vi "VisualizePMU.vi"() -> ()   [LabVIEW 2017, in "Visualization.lvlib" / "VisualizePMU_class.lvclass"]
uses:
  VisualizePMU_class.lvclass
  Framework/Bus_class/Bus.lvclass
  VisializeBase_class/Typedefs/VisualizeData.ctl
  VisializeBase_class/Typedefs/clVisualizeData.ctl
  Modules/EventPlugins/EventPluginBaseClass/TypeDefs/clEvtReportArray.ctl
  Modules/EventPlugins/EventPluginBaseClass/TypeDefs/clEvtReport.ctl
  Modules/EventPlugins/EventPluginBaseClass/TypeDefs/dblEvtSignalArray.ctl
  Modules/NetworkImpairmentModule/PublicAPI/Arguments/Broadcasts/dblNetworkTime.ctl
  Modules/NetworkImpairmentModule/PublicAPI/Arguments/Broadcasts/dblPktLoss.ctl
  Modules/FlagImpairModule/PublicAPI/Arguments/Broadcasts/ui32FlagImpairmentArray.ctl
  Framework/Bus_class/Broadcast/Typedefs/clDidInit.ctl
  QMH/Typedefs/clEvtRptArray.ctl
  QMH/Typedefs/clEvtRptSignal.ctl
  QMH/Typedefs/clPmuImpairRptArray.ctl
  VisializeBase_class/Requests/clUserEventType.ctl
  <vilib>/event_ctls.llb/usereventprio.ctl
  <vilib>/Utility/miscctls.llb/LVStringsAndValuesArrayTypeDef_U8.ctl
  QMH/Typedefs/clNetImpairmentTime.ctl
  QMH/Typedefs/clNetIPktLoss.ctl
  QMH/Typedefs/clFlagImpairArray.ctl
  <vilib>/Utility/error.llb/Error Cluster From Error Code.vi
  <vilib>/ErrorRing/Error Ring.xnode
  VisializeBase_class/VisualizeBase_class.lvclass
  <userlib>/NIST/NISTErrorLib/NISTErrorLib.lvlib
  Framework/Bus_class/Bus_class.lvlib
  Modules/EventModule/EventModule.lvlib
  Modules/PmuImpairModule/PmuImpairModule.lvlib
  Modules/NetworkImpairmentModule/NetworkImpairmentModule.lvlib
  Modules/FlagImpairModule/FlagImpairModule.lvlib
  Modules/EventPlugins/EventPluginBaseClass/EventPluginBaseClass.lvclass
  VisualizeApp_class/VisualizeAppBase_class.lvclass
panel:
  in  "QueName":string="VisPmuQue"
  out "RFE Plot":cluster{dbl[], "TVE":dbl[]}[](graph)
  out "FE Plot":cluster{dbl[], "TVE":dbl[]}[](graph)
  out "PE Plot":cluster{dbl[], "TVE":dbl[]}[](graph)
  out "Mag Error":cluster{dbl[], "TVE":dbl[]}[](graph)
  out "TVE Plot":cluster{dbl[], "TVE":dbl[]}[](graph)
  in  "Bus Number":u8(ring)
  out "ErrorArray":errorcluster[](array[cluster])
  in  "btnStop":bool
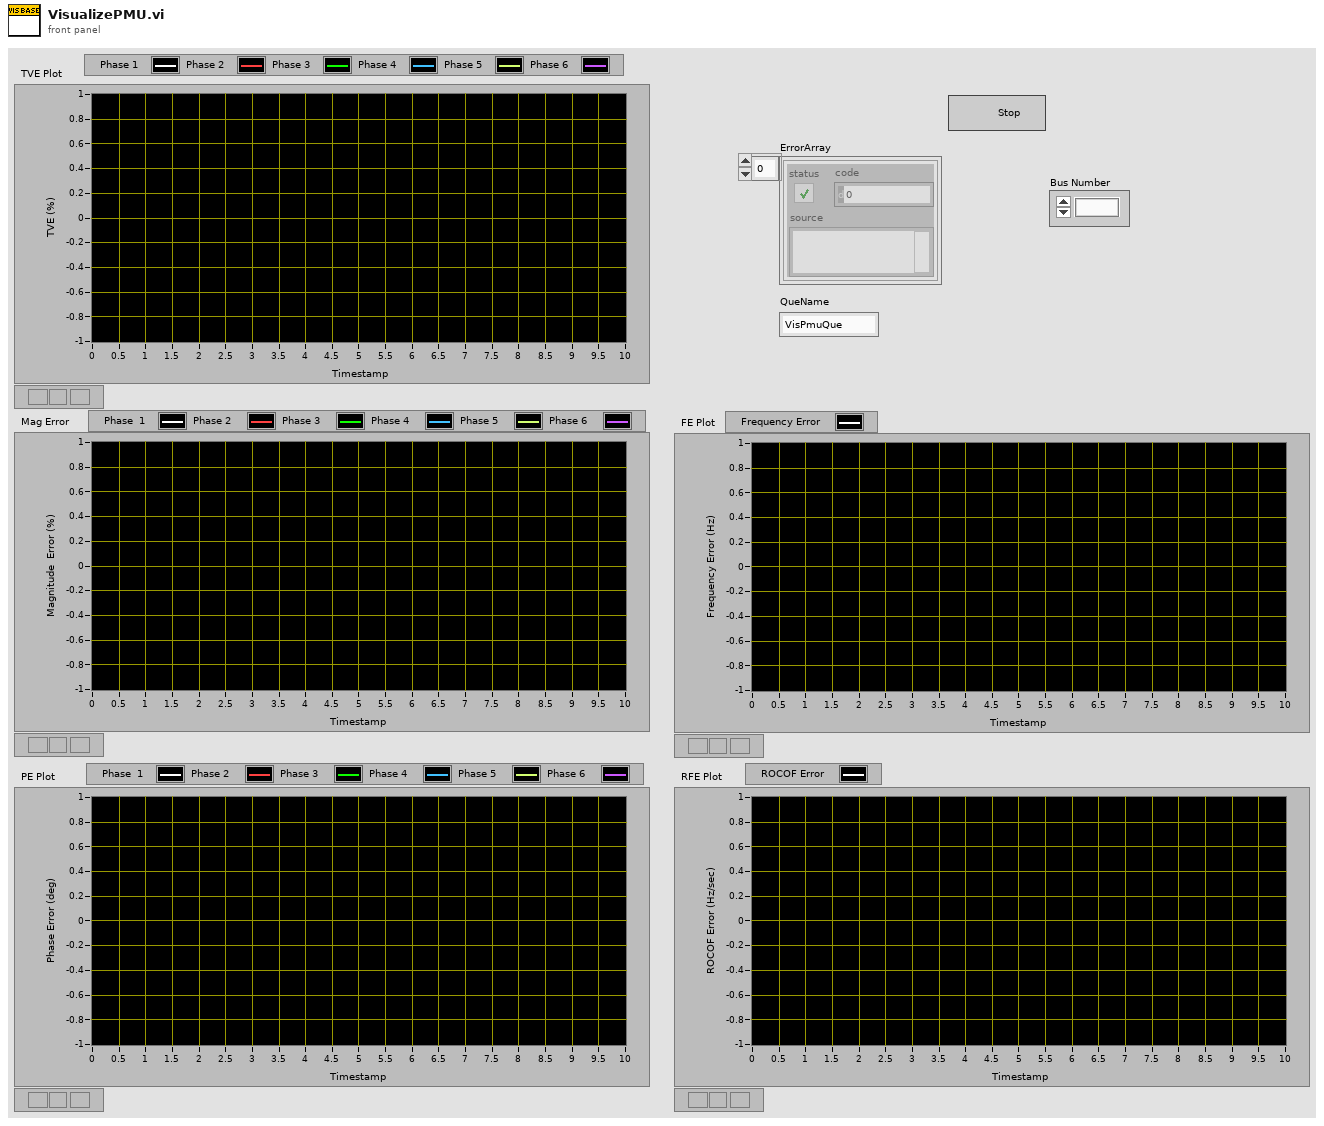
[diagram p1: front panel]
types:
  T1 = typedef "Visualization.lvlib/VisualizeBase_class.lvclass/VisualizeData.ctl" = T2[]
  T2 = typedef "Visualization.lvlib/VisualizeAppBase_class.lvclass/clVisualizeData.ctl" = cluster{"clEvtReportArray":T3, "dblEventSignalArray":T5, "clPmuImpairRptArray":T3, "dblNetworkTime":T6, "dblPktLoss":T7, "FlagImpairArray":T8, "TimeArray":dbl[]}
  T3 = typedef "EventPlugins.lvlib/EventPluginBaseClass.lvclass/clEvtReportArray.ctl" = T4[]
  T4 = typedef "EventPlugins.lvlib/EventPluginBaseClass.lvclass/clEvtReport.ctl" = cluster{"Timestamp":dbl, "Synx":cdb[], "Freq":dbl, "ROCOF":dbl, "ID":i16}
  T5 = typedef "EventPlugins.lvlib/EventPluginBaseClass.lvclass/dblEvtSignalArray.ctl" = dbl[][]
  T6 = typedef "NetworkImpairmentModule.lvlib/dblNetworkTime.ctl" = dbl[]
  T7 = typedef "NetworkImpairmentModule.lvlib/dblPktLoss.ctl" = dbl[]
  T8 = typedef "FlagImpairModule.lvlib/ui32FlagImpairmentArray.ctl" = u32[]
  T9 = typedef "Visualization.lvlib/VisualizeBase_class.lvclass/clRequestEvents.ctl" = cluster{"StopRequest":refnum<user-event>}
  T10 = typedef "Bus_class.lvlib/clBroadcastEvents.ctl" = cluster{"DidInit":refnum<user-event>, "DidStop":refnum<user-event>}
  T11 = typedef "EventModule.lvlib/clBroadcastEvents.ctl" = cluster{"DidInit":refnum<user-event>, "StatusUpdate":refnum<user-event>, "ErrorReport":refnum<user-event>, "DidStop":refnum<user-event>, "ReadEvtConfig":refnum<user-event>, "ReadTimeArray":refnum<user-event>, "ReadEvtParams":refnum<user-event>, "GetEvtReportArray":refnum<user-event>, "ReadPathToPlugin":refnum<user-event>, "GetEvtSignal":refnum<user-event>, "ReadBusNumber":refnum<user-event>}
  T12 = typedef "PmuImpairModule.lvlib/clBroadcastEvents.ctl" = cluster{"DidInit":refnum<user-event>, "StatusUpdate":refnum<user-event>, "ErrorReport":refnum<user-event>, "DidStop":refnum<user-event>, "ImpairConfig":refnum<user-event>, "ImpairParams":refnum<user-event>, "ImpairReports":refnum<user-event>, "PathToPlugin":refnum<user-event>, "BusNumber":refnum<user-event>}
  T13 = typedef "NetworkImpairmentModule.lvlib/clBroadcastEvents.ctl" = cluster{"DidInit":refnum<user-event>, "StatusUpdate":refnum<user-event>, "ErrorReport":refnum<user-event>, "DidStop":refnum<user-event>, "ReadNetImpParams":refnum<user-event>, "ReadLossThreshold":refnum<user-event>, "GetNetworkTime":refnum<user-event>, "GetPktLoss":refnum<user-event>, "ReadPathToPlugin":refnum<user-event>}
  T14 = typedef "FlagImpairModule.lvlib/clBroadcastEvents.ctl" = cluster{"DidInit":refnum<user-event>, "StatusUpdate":refnum<user-event>, "ErrorReport":refnum<user-event>, "DidStop":refnum<user-event>, "ReadFlagImpairConfig":refnum<user-event>, "ReadPluginINIFilePath":refnum<user-event>, "ReadFlagImpairParams":refnum<user-event>, "ReadTimeArray":refnum<user-event>, "GetFlagImpairment":refnum<user-event>}
  T15 = cluster{"BusNumberRef":refnum<vi>, "TVE Plot":refnum<vi>, "Mag Error":refnum<vi>, "PE Plot":refnum<vi>, "FE Plot":refnum<vi>, "RFE Plot":refnum<vi>}
  T16 = typedef "LVStringsAndValuesArrayTypeDef_U8.ctl" = cluster{"String":string, "Value":u8}[]
  T17 = typedef "Visualization.lvlib/VisualizeBase_class.lvclass/clEvtRptArray.ctl" = cluster{"BusIndex":i32, "clImpairReportArray":T3}
  T18 = typedef "Visualization.lvlib/VisualizeBase_class.lvclass/clPmuImpairRptArray.ctl" = cluster{"BusIndex":i32, "clImpairReportArray":T3}
  T19 = typedef "Visualization.lvlib/VisualizeBase_class.lvclass/clNetImpairmentTime.ctl" = cluster{"BusIndex":i32, "clNetImpairTimeArray":T6}
  T20 = typedef "Visualization.lvlib/VisualizeBase_class.lvclass/clNetIPktLoss.ctl" = cluster{"BusIndex":i32, "clNetPktLoss":T7}
  T21 = typedef "Visualization.lvlib/VisualizeBase_class.lvclass/clFlagImpairArray.ctl" = cluster{"BusIndex":i32, "FlagImpairArray":T8}
  T22 = typedef "Visualization.lvlib/VisualizeBase_class.lvclass/clEvtRptSignal.ctl" = cluster{"BusIndex":i32, "dblEventSignalArray":T5}
  T23 = typedef "Visualization.lvlib/VisualizeBase_class.lvclass/clUserEventType.ctl" = cluster{"BusIndex":i8, "Data":variant}
  T24 = typedef "usereventprio.ctl" = enum32{"high priority", "normal priority"}
  T25 = typedef "Bus_class.lvlib/clDidInit.ctl" = cluster{"Bus":refnum<vi>, "Init?":bool}
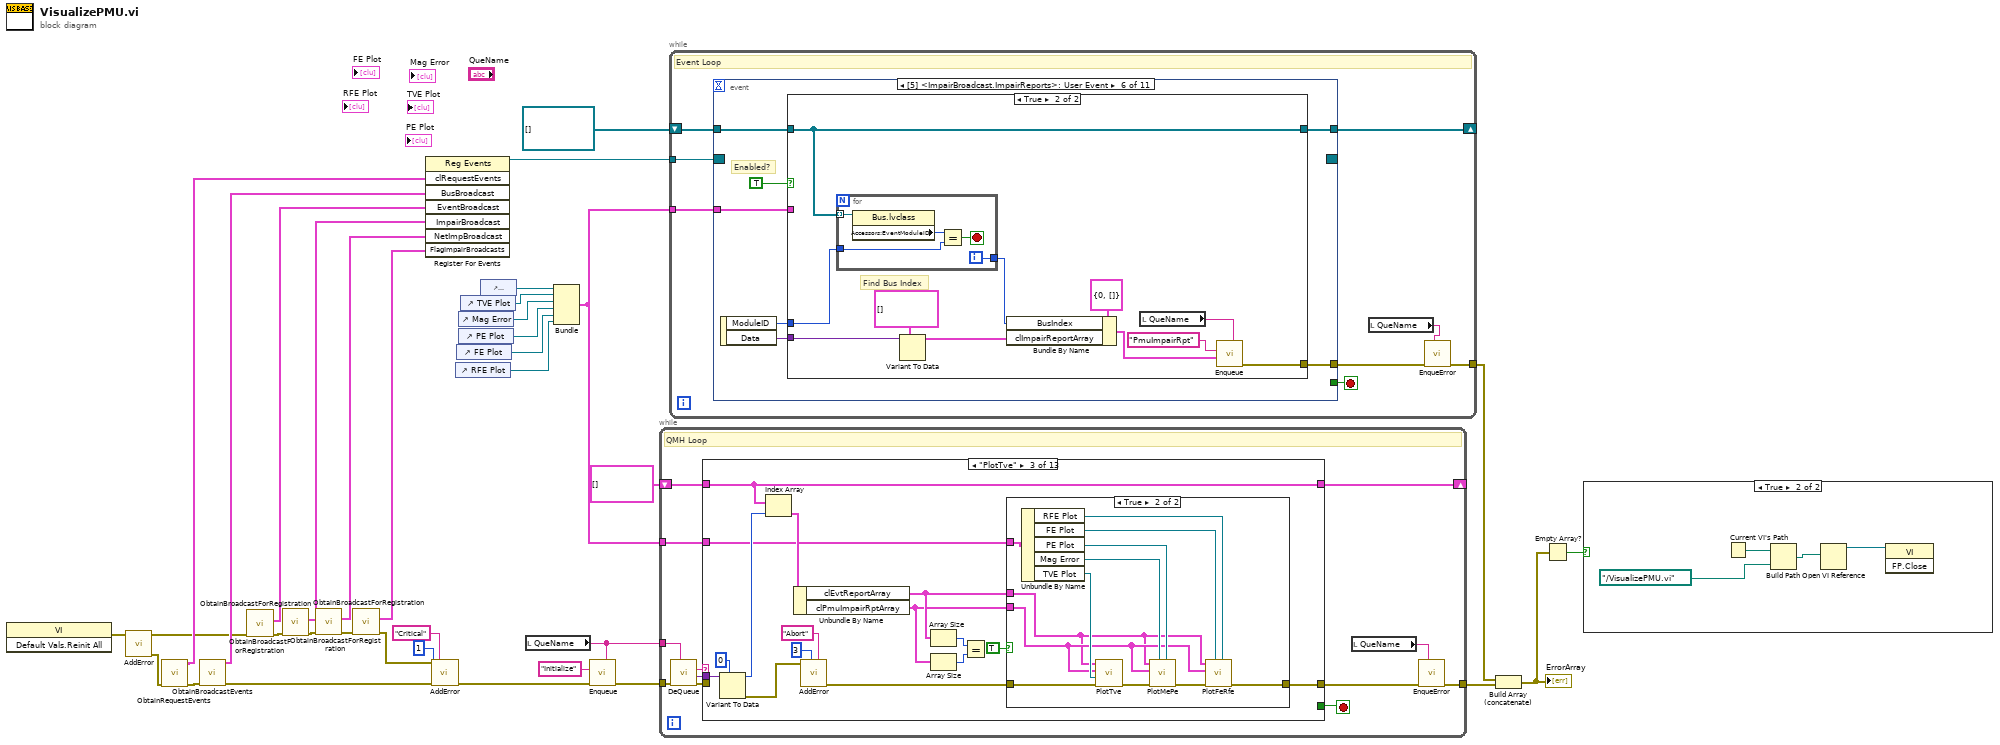
[diagram p0: block diagram]
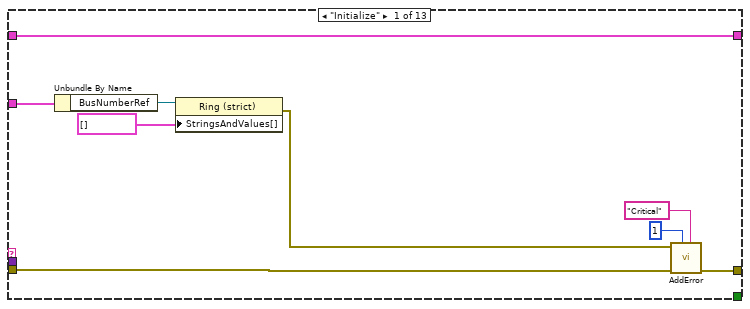
[diagram p3: hidden frame]
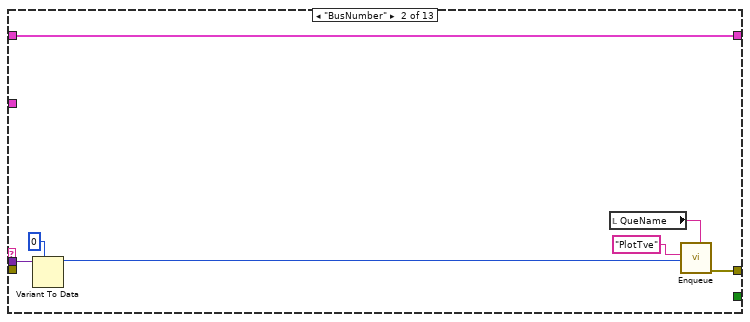
[diagram p4: hidden frame]
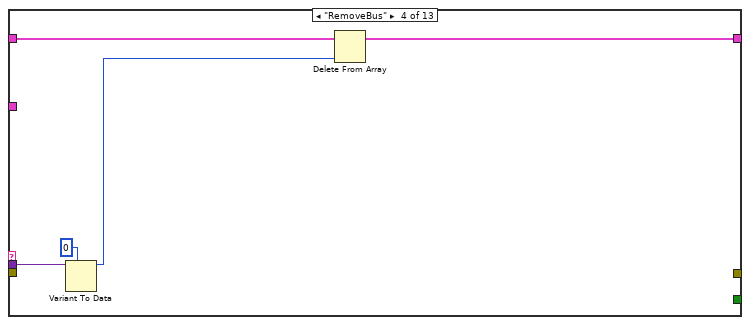
[diagram p6: hidden frame]
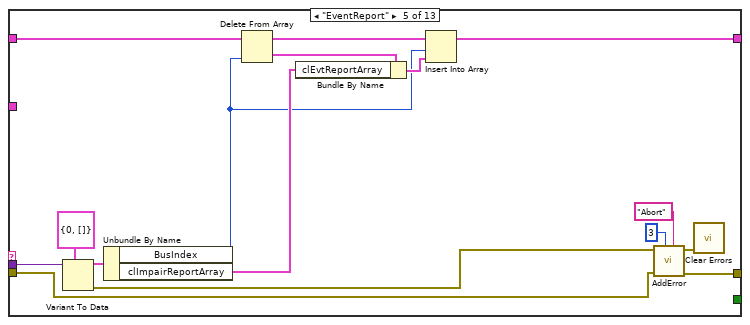
[diagram p7: hidden frame]
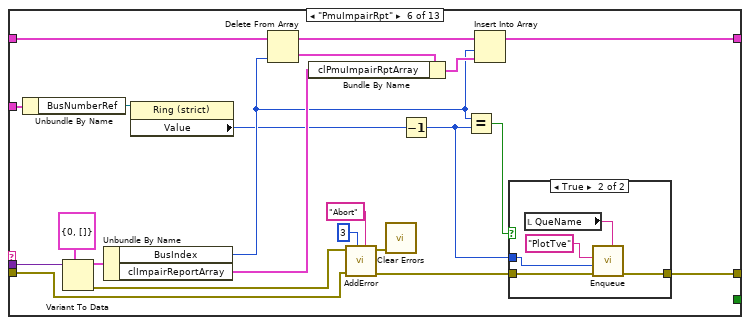
[diagram p8: hidden frame]
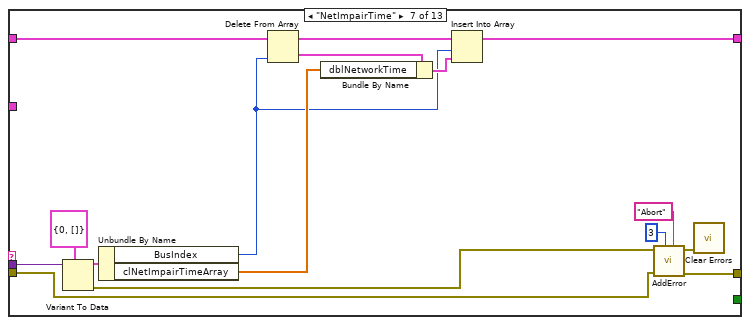
[diagram p10: hidden frame]
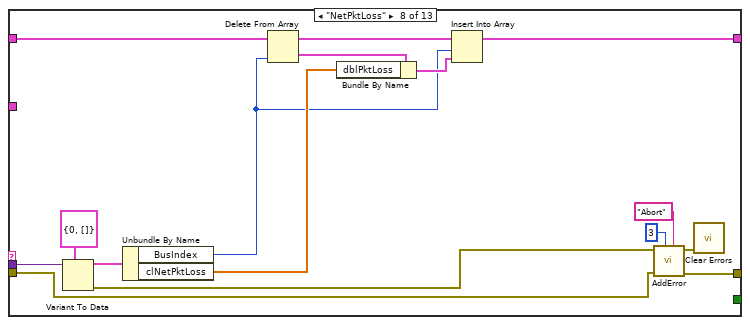
[diagram p11: hidden frame]
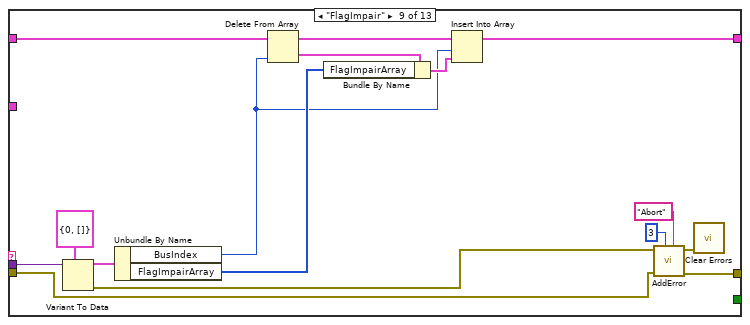
[diagram p12: hidden frame]
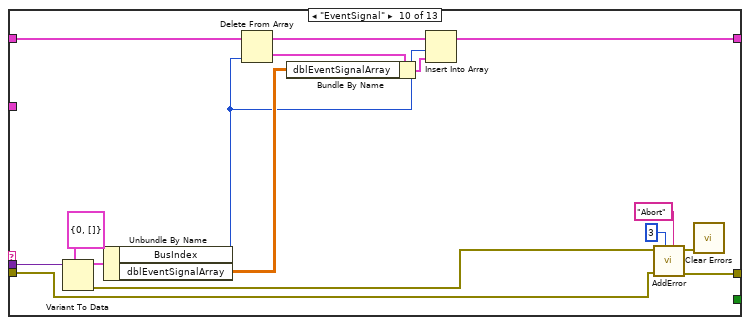
[diagram p13: hidden frame]
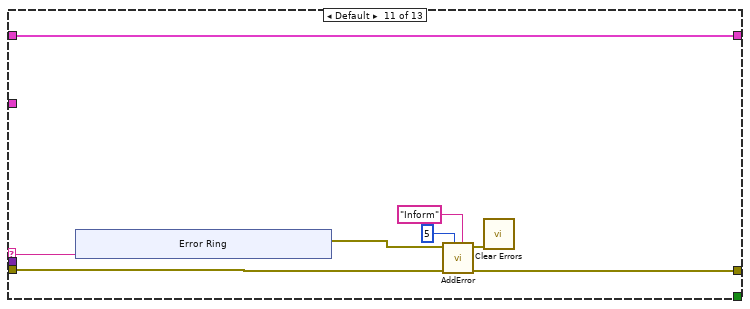
[diagram p14: hidden frame]
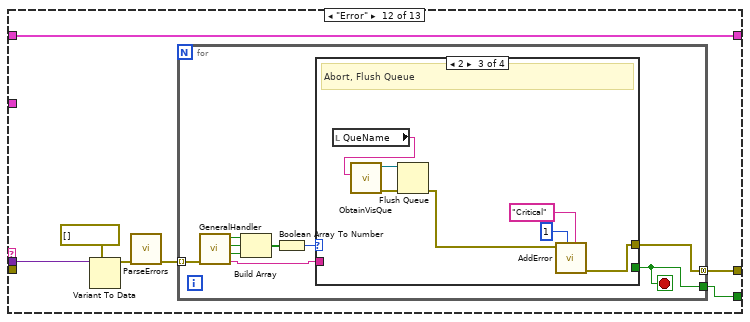
[diagram p15: hidden frame]
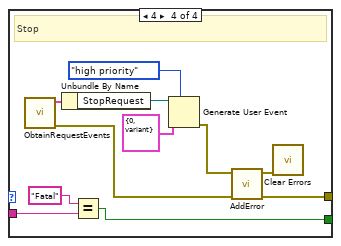
[diagram p18: hidden frame]
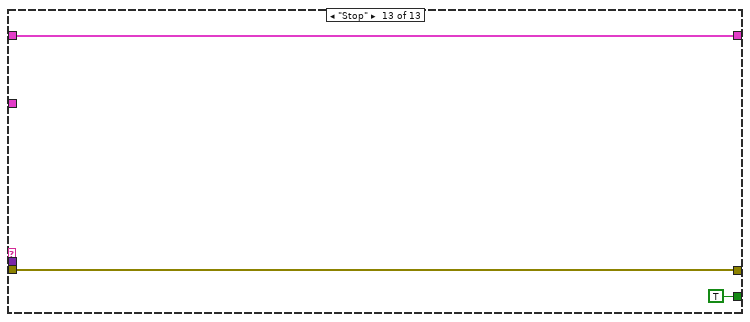
[diagram p19: hidden frame]
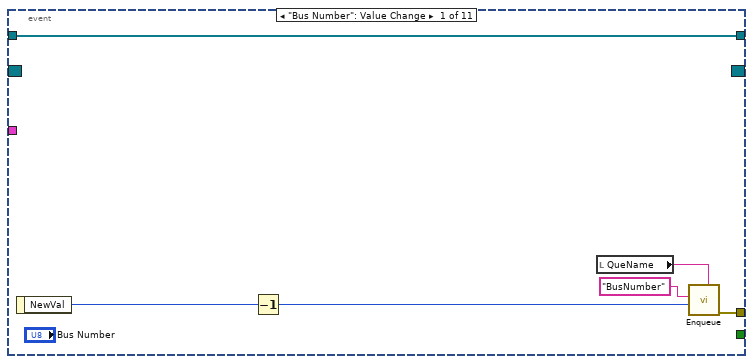
[diagram p20: hidden frame]
diagram:
  n1 = invoke class="VI" method="Default Vals.Reinit All"() -> (error out=w25:errorcluster)  [unwired: 3 in, 2 out]
  n2 = call <userlib>:"AddError.vi"("error in (no error)"=w25) -> ("ErrorArray"=w24:errorcluster[], "error out"=w16:errorcluster)  [unwired: 9 in]
  n3 = call "ObtainRequestEvents.vi"("Error"=w24) -> ("Error"=w29:errorcluster[], "clRequestEvents"=w33:T9)  [unwired: 9 in]
  n4 = call "ObtainBroadcastEvents.vi"("ErrorArray"=w29) -> ("ErrorArray"=w15:errorcluster[], "BusBroadcast"=w28:T10)  [unwired: 9 in]
  n5 = call "ObtainBroadcastForRegistration.vi"("error in (no error)"=w16) -> ("error out"=w19:errorcluster, "EventBroadcast"=w23:T11)  [unwired: 9 in]
  n6 = call "ObtainBroadcastForRegistration.vi"("error in (no error)"=w19) -> ("error out"=w18:errorcluster, "ImpairBroadcast"=w22:T12)  [unwired: 9 in]
  n7 = call "ObtainBroadcastForRegistration.vi"("error in (no error)"=w18) -> ("error out"=w17:errorcluster, "NetImpBroadcast"=w21:T13)  [unwired: 9 in]
  n8 = call "ObtainBroadcastForRegistration.vi"("error in (no error)"=w17) -> ("error out"=w14:errorcluster, "FlagImpairBroadcasts"=w20:T14)  [unwired: 9 in]
  n9 = register-events(w33, w28, w23, w22, w21, w20) -> (reference out=w32:refnum<event-registration>)  [unwired: 2 in, 1 out]
  n10 = call <userlib>:"AddError.vi"("Severity"="Critical" ("String"), "Priority"=u8 1, "ErrorArray"=w15, "error in (no error)"=w14) -> ("ErrorArray"=w11:errorcluster[])  [unwired: 6 in, 1 out]
  n11 = control-ref of="RFE Plot"() -> (w4:refnum<vi>)
  n12 = control-ref of="FE Plot"() -> (w5:refnum<vi>)
  n13 = control-ref of="PE Plot"() -> (w6:refnum<vi>)
  n14 = control-ref of="Mag Error"() -> (w7:refnum<vi>)
  n15 = control-ref of="TVE Plot"() -> (w8:refnum<vi>)
  n16 = control-ref of="BusNumberRef"() -> (w27:refnum<vi>)
  n17 = local read "QueName"() -> (w3:string)
  n18 = Bundle("BusNumberRef"=w27, "TVE Plot"=w8, "Mag Error"=w7, "PE Plot"=w6, "FE Plot"=w5, "RFE Plot"=w4) -> (w9:T15)  [unwired: 1 in]
  n19 = call "Enqueue.vi"("QueName"=w3, "Error"=w11, "Message"="Initialize") -> ("Error"=w34:errorcluster[])  [unwired: 8 in]
  n20 = while {
    tunnel: w34 -> [w47]
    tunnel: [w41] -> w31
    tunnel: w9 -> [w40]
    shift-right: [w38] -> _
    shift-left: T1 [] ("VisualizeData") -> [w39]
    tunnel: w3 -> [w36]
    stop <- w42 stop-if-true
    # "QMH Loop"
    n21 = call "DeQueue.vi"("QueName"=w36, "Error"=w47) -> ("Error"=w44:errorcluster[], "Data"=w45:variant, "Message"=w46:string)  [unwired: 7 in]
    n22 = case shown="\"PlotTve\"" w46 {
      selector: w46 -> [_ _ _ _ _ _ _ _ _ _ w212 _ _]
      tunnel: w45 -> [_ w61 w79 w96 w112 w134 w156 w172 w188 w204 _ w226 _]
      tunnel: w44 -> [w53 _ _ _ w97 w121 w141 w157 w173 w189 w210 _ w255]
      tunnel: [w52 w63 w69 _ w102 w119 w146 w162 w178 w194 w209 w222 w255] -> w43
      tunnel: [_ _ _ _ _ _ _ _ _ _ _ w221 TRUE] -> w42
      tunnel: w40 -> [w56 _ w72 _ _ w118 _ _ _ _ _ _ _]
      tunnel: w39 -> [w48 w58 w77 w94 w108 w130 w152 w168 w184 w200 w205 w220 w254]
      tunnel: [w48 w58 w77 w93 w109 w131 w153 w169 w185 w201 w205 w220 w254] -> w38
      frame "Initialize" {
        n23 = Unbundle By Name(w56) -> ("BusNumberRef"=w55:refnum<vi>)
        n24 = property class="Ring (strict)"(reference=w55, "StringsAndValues[]"=T16 [] ("Strings And Values []")) -> (error out=w51:errorcluster)  [unwired: 1 in, 1 out]
        n25 = call <userlib>:"AddError.vi"("Severity"="Critical" ("String"), "Priority"=u8 1, "ErrorArray"=w53, "error in (no error)"=w51) -> ("ErrorArray"=w52:errorcluster[])  [unwired: 6 in, 1 out]
      }
      frame "BusNumber" {
        n26 = Variant To Data(type=u8 0 ("NewVal"), Variant=w61) -> (data=w60:u8)  [unwired: 1 in, 1 out]
        n27 = local read "QueName"() -> (w57:string)
        n28 = call "Enqueue.vi"("QueName"=w57, "Data"=w60, "Message"="PlotTve") -> ("Error"=w63:errorcluster[])  [unwired: 8 in]
      }
      frame "PlotTve" {
        n29 = Variant To Data(type=u8 0 ("NewVal"), Variant=w79) -> (data=w76:u8, error out=w68:errorcluster)  [unwired: 1 in]
        n30 = Index Array(array=w77, index=w76) -> (element=w75:T2)
        n31 = Unbundle By Name(w75) -> ("clEvtReportArray"=w71:T3, "clPmuImpairRptArray"=w70:T3)
        n32 = call <userlib>:"AddError.vi"("Severity"="Abort" ("String"), "Priority"=u8 3, "error in (no error)"=w68) -> ("ErrorArray"=w67:errorcluster[])  [unwired: 7 in, 1 out]
        n33 = Array Size(array=w71) -> (size(s)=w73:i32)
        n34 = Array Size(array=w70) -> (size(s)=w74:i32)
        n35 = Equal?(x=w73, y=w74) -> ()  [unwired: 1 out]
        n36 = case shown="True" TRUE {
          tunnel: w72 -> [_ w91]
          tunnel: w71 -> [_ w82]
          tunnel: w70 -> [_ w83]
          tunnel: [_ w84] -> w69
          tunnel: w67 -> [_ w89]
          frame False {
          }
          frame True {
            n37 = Unbundle By Name(w91) -> ("RFE Plot"=w80:refnum<vi>, "FE Plot"=w81:refnum<vi>, "PE Plot"=w86:refnum<vi>, "Mag Error"=w87:refnum<vi>, "TVE Plot"=w90:refnum<vi>)
            n38 = call "PlotTve.vi"("ErrorArray"=w89, "TvePlotRef"=w90, "clPMUImpairRptArray"=w83, "clEvtReportArray"=w82) -> ("ErrorArray"=w88:errorcluster[])  [unwired: 7 in]
            n39 = call "PlotMePe.vi"("PePlotRef"=w86, "MePlotRef"=w87, "ErrorArray"=w88, "clPmuRptArray"=w83, "clEvtReportArray"=w82) -> ("ErrorArray"=w85:errorcluster[])  [unwired: 6 in]
            n40 = call "PlotFeRfe.vi"("REPlotRef"=w80, "FEPlotRef"=w81, "ErrorArray"=w85, "clPmuImpairRptArray"=w83, "clEvtReportArray"=w82) -> ("ErrorArray"=w84:errorcluster[])  [unwired: 6 in]
          }
        }
      }
      frame "RemoveBus" {
        n41 = Variant To Data(type=0, Variant=w96) -> (data=w92:i32)  [unwired: 1 in, 1 out]
        n42 = Delete From Array(array=w94, index=w92) -> (array with subset deleted=w93:T1)  [unwired: 1 in, 1 out]
      }
      frame "EventReport" {
        n43 = Variant To Data(type=T17 {"BusIndex"=0, "clImpairReportArray"=[]} ("clEvtReportArray"), Variant=w112) -> (data=w110:T17, error out=w101:errorcluster)  [unwired: 1 in]
        n44 = Unbundle By Name(w110) -> ("BusIndex"=w103:i32, "clImpairReportArray"=w105:T3)
        n45 = Delete From Array(array=w108, index=w103) -> (deleted portion=w106:T2, array with subset deleted=w107:T1)  [unwired: 1 in]
        n46 = Bundle By Name(cluster=w106, "clEvtReportArray"=w105) -> (w104:T2)
        n47 = Insert Into Array(array=w107, index=w103, new element=w104) -> (w109:T1)
        n48 = call <userlib>:"AddError.vi"("Severity"="Abort" ("String"), "Priority"=u8 3, "ErrorArray"=w97, "error in (no error)"=w101) -> ("ErrorArray"=w102:errorcluster[], "error out"=w100:errorcluster)  [unwired: 6 in]
        n49 = call <vilib>:"Clear Errors.vi"("error in (no error)"=w100) -> ()  [unwired: 5 in, 2 out]
      }
      frame "PmuImpairRpt" {
        n50 = Unbundle By Name(w118) -> ("BusNumberRef"=w117:refnum<vi>)
        n51 = Variant To Data(type=T18 {"BusIndex"=0, "clImpairReportArray"=[]} ("clImpairReportArray"), Variant=w134) -> (data=w132:T18, error out=w125:errorcluster)  [unwired: 1 in]
        n52 = Unbundle By Name(w132) -> ("BusIndex"=w116:i32, "clImpairReportArray"=w127:T3)
        n53 = property class="Ring (strict)"(reference=w117) -> ("Value"=w114:u8)  [unwired: 1 in, 2 out]
        n54 = Delete From Array(array=w130, index=w116) -> (deleted portion=w128:T2, array with subset deleted=w129:T1)  [unwired: 1 in]
        n55 = Bundle By Name(cluster=w128, "clPmuImpairRptArray"=w127) -> (w126:T2)
        n56 = call <userlib>:"AddError.vi"("Severity"="Abort" ("String"), "Priority"=u8 3, "ErrorArray"=w121, "error in (no error)"=w125) -> ("ErrorArray"=w120:errorcluster[], "error out"=w124:errorcluster)  [unwired: 6 in]
        n57 = call <vilib>:"Clear Errors.vi"("error in (no error)"=w124) -> ()  [unwired: 5 in, 2 out]
        n58 = Decrement(x=w114) -> (x-1=w113:u8)
        n59 = Equal?(x=w116, y=w113) -> (x = y?=w115:bool)
        n60 = Insert Into Array(array=w129, index=w116, new element=w126) -> (w131:T1)
        n61 = case shown="True" w115 {
          tunnel: w120 -> [w135 w140]
          tunnel: [w135 w139] -> w119
          tunnel: w113 -> [_ w137]
          frame False {
          }
          frame True {
            n62 = local read "QueName"() -> (w136:string)
            n63 = call "Enqueue.vi"("QueName"=w136, "Error"=w140, "Data"=w137, "Message"="PlotTve") -> ("Error"=w139:errorcluster[])  [unwired: 7 in]
          }
        }
      }
      frame "NetImpairTime" {
        n64 = Variant To Data(type=T19 {"BusIndex"=0, "clNetImpairTimeArray"=[]} ("clImpairReportArray"), Variant=w156) -> (data=w154:T19, error out=w145:errorcluster)  [unwired: 1 in]
        n65 = Unbundle By Name(w154) -> ("BusIndex"=w147:i32, "clNetImpairTimeArray"=w149:T6)
        n66 = Delete From Array(array=w152, index=w147) -> (deleted portion=w150:T2, array with subset deleted=w151:T1)  [unwired: 1 in]
        n67 = Bundle By Name(cluster=w150, "dblNetworkTime"=w149) -> (w148:T2)
        n68 = Insert Into Array(array=w151, index=w147, new element=w148) -> (w153:T1)
        n69 = call <userlib>:"AddError.vi"("Severity"="Abort" ("String"), "Priority"=u8 3, "ErrorArray"=w141, "error in (no error)"=w145) -> ("ErrorArray"=w146:errorcluster[], "error out"=w144:errorcluster)  [unwired: 6 in]
        n70 = call <vilib>:"Clear Errors.vi"("error in (no error)"=w144) -> ()  [unwired: 5 in, 2 out]
      }
      frame "NetPktLoss" {
        n71 = Variant To Data(type=T20 {"BusIndex"=0, "clNetPktLoss"=[]} ("clNetPktLoss"), Variant=w172) -> (data=w170:T20, error out=w161:errorcluster)  [unwired: 1 in]
        n72 = Unbundle By Name(w170) -> ("BusIndex"=w163:i32, "clNetPktLoss"=w165:T7)
        n73 = Delete From Array(array=w168, index=w163) -> (deleted portion=w166:T2, array with subset deleted=w167:T1)  [unwired: 1 in]
        n74 = Bundle By Name(cluster=w166, "dblPktLoss"=w165) -> (w164:T2)
        n75 = Insert Into Array(array=w167, index=w163, new element=w164) -> (w169:T1)
        n76 = call <userlib>:"AddError.vi"("Severity"="Abort" ("String"), "Priority"=u8 3, "ErrorArray"=w157, "error in (no error)"=w161) -> ("ErrorArray"=w162:errorcluster[], "error out"=w160:errorcluster)  [unwired: 6 in]
        n77 = call <vilib>:"Clear Errors.vi"("error in (no error)"=w160) -> ()  [unwired: 5 in, 2 out]
      }
      frame "FlagImpair" {
        n78 = Variant To Data(type=T21 {"BusIndex"=0, "FlagImpairArray"=[]} ("clFlagImpairArray"), Variant=w188) -> (data=w186:T21, error out=w177:errorcluster)  [unwired: 1 in]
        n79 = Unbundle By Name(w186) -> ("BusIndex"=w179:i32, "FlagImpairArray"=w181:T8)
        n80 = Delete From Array(array=w184, index=w179) -> (deleted portion=w182:T2, array with subset deleted=w183:T1)  [unwired: 1 in]
        n81 = Bundle By Name(cluster=w182, "FlagImpairArray"=w181) -> (w180:T2)
        n82 = Insert Into Array(array=w183, index=w179, new element=w180) -> (w185:T1)
        n83 = call <userlib>:"AddError.vi"("Severity"="Abort" ("String"), "Priority"=u8 3, "ErrorArray"=w173, "error in (no error)"=w177) -> ("ErrorArray"=w178:errorcluster[], "error out"=w176:errorcluster)  [unwired: 6 in]
        n84 = call <vilib>:"Clear Errors.vi"("error in (no error)"=w176) -> ()  [unwired: 5 in, 2 out]
      }
      frame "EventSignal" {
        n85 = Variant To Data(type=T22 {"BusIndex"=0, "dblEventSignalArray"=[]} ("clEvtReportArray"), Variant=w204) -> (data=w202:T22, error out=w193:errorcluster)  [unwired: 1 in]
        n86 = Unbundle By Name(w202) -> ("BusIndex"=w195:i32, "dblEventSignalArray"=w197:T5)
        n87 = Delete From Array(array=w200, index=w195) -> (deleted portion=w198:T2, array with subset deleted=w199:T1)  [unwired: 1 in]
        n88 = Bundle By Name(cluster=w198, "dblEventSignalArray"=w197) -> (w196:T2)
        n89 = Insert Into Array(array=w199, index=w195, new element=w196) -> (w201:T1)
        n90 = call <userlib>:"AddError.vi"("Severity"="Abort" ("String"), "Priority"=u8 3, "ErrorArray"=w189, "error in (no error)"=w193) -> ("ErrorArray"=w194:errorcluster[], "error out"=w192:errorcluster)  [unwired: 6 in]
        n91 = call <vilib>:"Clear Errors.vi"("error in (no error)"=w192) -> ()  [unwired: 5 in, 2 out]
      }
      frame Default {
        n92 = xnode "Error Ring"("parameter 0"=w212) -> ("error out"=w211:errorcluster)
        n93 = call <userlib>:"AddError.vi"("Severity"="Inform" ("String"), "Priority"=u8 5, "ErrorArray"=w210, "error in (no error)"=w211) -> ("ErrorArray"=w209:errorcluster[], "error out"=w208:errorcluster)  [unwired: 6 in]
        n94 = call <vilib>:"Clear Errors.vi"("error in (no error)"=w208) -> ()  [unwired: 5 in, 2 out]
      }
      frame "Error" {
        n95 = Variant To Data(type=errorcluster[] [], Variant=w226) -> (data=w224:errorcluster[])  [unwired: 1 in, 1 out]
        n96 = call <userlib>:"ParseErrors.vi"("ErrorArray"=w224) -> ("ErrorArray"=w223:errorcluster[])  [unwired: 8 in, 2 out]
        n97 = for {
          tunnel: w223 -> [w235] mode=indexing
          tunnel: [w229] -> w222 mode=concatenating
          tunnel: [w227] -> w221
          stop <- w227 stop-if-true
          n98 = call <userlib>:"GeneralHandler.vi"("error in (no error)"=w235) -> ("Severity"=w228:string, "Stop"=w232:bool, "Abort"=w233:bool, "Continue"=w234:bool)  [unwired: 7 in]
          n99 = Build Array(w234, w233, w232) -> (w231:bool[])
          n100 = Boolean Array To Number(Boolean array=w231) -> (number=w230:u32)
          n101 = case shown="2" w230 {
            tunnel: [_ _ w240 w251] -> w229
            tunnel: w228 -> [_ _ _ w245]
            tunnel: [_ _ _ w243] -> w227
            frame 0, Default {
              # "No Dialog"
            }
            frame 1 {
              # "Continue"
            }
            frame 2 {
              # "Abort, Flush Queue"
              n102 = local read "QueName"() -> (w236:string)
              n103 = call "ObtainVisQue.vi"("QueName"=w236) -> ("error out"=w242:errorcluster, "queue out"=w241:refnum<queue>)  [unwired: 9 in]
              n104 = Flush Queue(queue=w241, error in (no error)=w242) -> (error out=w239:errorcluster)  [unwired: 2 out]
              n105 = call <userlib>:"AddError.vi"("Severity"="Critical" ("String"), "Priority"=u8 1, "error in (no error)"=w239) -> ("ErrorArray"=w240:errorcluster[])  [unwired: 7 in, 1 out]
            }
            frame 4 {
              # "Stop"
              n106 = call "ObtainRequestEvents.vi"() -> ("Error"=w249:errorcluster[], "clRequestEvents"=w253:T9)  [unwired: 10 in]
              n107 = Unbundle By Name(w253) -> ("StopRequest"=w252:refnum<user-event>)
              n108 = Equal?(x="Fatal", y=w245) -> (x = y?=w243:bool)
              n109 = Generate User Event(priority (normal)=usereventprio."high priority", user event=w252, event data cluster=T23 {"BusIndex"=0, "Data"=variant} ("event data")) -> (error out=w250:errorcluster)  [unwired: 1 in, 1 out]
              n110 = call <userlib>:"AddError.vi"("ErrorArray"=w249, "error in (no error)"=w250) -> ("ErrorArray"=w251:errorcluster[], "error out"=w246:errorcluster)  [unwired: 8 in]
              n111 = call <vilib>:"Clear Errors.vi"("error in (no error)"=w246) -> ()  [unwired: 5 in, 2 out]
            }
          }
        }
      }
      frame "Stop" {
      }
    }
    n112 = local read "QueName"() -> (w37:string)
    n113 = call "EnqueError.vi"("QueName"=w37, "Error"=w43) -> ("Error"=w41:errorcluster[])  [unwired: 9 in]
  }
  n114 = while {
    tunnel: w32 -> [w264]
    tunnel: [w261] -> w30
    tunnel: w9 -> [w260]
    shift-right: [w258] -> _
    shift-left: refnum<class "Bus.lvclass">[] [] -> [w259]
    stop <- w263 stop-if-true
    # "Event Loop"
    n115 = event shown="[5] <ImpairBroadcast.ImpairReports>: User Event" {
      selector: w264 -> [_ _ _ _ _ _ _ _ _ _ _]
      dyn-events: [_ w271 _ _ _ _ _ _ _ _ _] -> _
      timeout: _ -> [_ _ _ _ _ _ _ _ _ _ _]
      tunnel: [_ _ _ _ _ _ _ _ _ TRUE _] -> w263
      tunnel: [w270 w272 w300 w307 w330 w354 w377 w400 w423 w448 w456] -> w262
      tunnel: w260 -> [_ w292 w304 _ _ w351 _ _ _ _ _]
      tunnel: w259 -> [w267 w291 w303 w310 w333 w357 w380 w403 w426 w445 w450]
      tunnel: [w267 w288 w302 w305 w328 w352 w375 w398 w421 w445 w450] -> w258
      event "Bus Number": Value Change {
        n116 = event-data() -> ("NewVal"=w269:u8)  [unwired: 1 in]
        n117 = Decrement(x=w269) -> (x-1=w265:u8)
        n118 = local read "QueName"() -> (w266:string)
        n119 = call "Enqueue.vi"("QueName"=w266, "Data"=w265, "Message"="BusNumber") -> ("Error"=w270:errorcluster[])  [unwired: 8 in]
      }
      event User Event {
        n120 = event-data() -> ("Data"=w295:variant)  [unwired: 1 in]
        n121 = Unbundle By Name(w292) -> ("BusNumberRef"=w290:refnum<vi>)
        n122 = Variant To Data(type=T25 {"Bus"=refnum, "Init?"=FALSE} ("clBusDidInit"), Variant=w295) -> (data=w293:T25)  [unwired: 1 in, 1 out]
        n123 = Unbundle By Name(w293) -> ("Bus"=w289:refnum<vi>)
        n124 = call "ObtainRequestEvents.vi"() -> ("Error"=w284:errorcluster[], "clRequestEvents"=w286:T9)  [unwired: 10 in]
        n125 = call "AddBus.vi"("BusRef"=w289, "BusNumberRef"=w290, "BusArray"=w291) -> ("BusArray"=w288:refnum<class "Bus.lvclass">[])  [unwired: 8 in]
        n126 = call "ObtainBroadcastEvents.vi"("ErrorArray"=w284) -> ("ErrorArray"=w285:errorcluster[], "BusBroadcast"=w287:T10)  [unwired: 9 in]
        n127 = call "ObtainBroadcastForRegistration.vi"() -> ("error out"=w273:errorcluster, "EventBroadcast"=w280:T11)  [unwired: 10 in]
        n128 = call "ObtainBroadcastForRegistration.vi"("error in (no error)"=w273) -> ("error out"=w274:errorcluster, "ImpairBroadcast"=w281:T12)  [unwired: 9 in]
        n129 = call "ObtainBroadcastForRegistration.vi"("error in (no error)"=w274) -> ("error out"=w275:errorcluster, "NetImpBroadcast"=w282:T13)  [unwired: 9 in]
        n130 = call "ObtainBroadcastForRegistration.vi"("error in (no error)"=w275) -> ("error out"=w279:errorcluster, "FlagImpairBroadcasts"=w283:T14)  [unwired: 9 in]
        n131 = register-events(w286, w287, w280, w281, w282, w283) -> (reference out=w271:refnum<event-registration>)  [unwired: 2 in, 1 out]
        n132 = call <userlib>:"AddError.vi"("Severity"="Critical" ("String"), "Priority"=u8 1, "ErrorArray"=w285, "error in (no error)"=w279) -> ("ErrorArray"=w272:errorcluster[], "error out"=w278:errorcluster)  [unwired: 6 in]
        n133 = call <vilib>:"Clear Errors.vi"("error in (no error)"=w278) -> ()  [unwired: 5 in, 2 out]
      }
      event User Event {
        n134 = event-data() -> ("BusNumber"=w297:i8)  [unwired: 1 in]
        n135 = Unbundle By Name(w304) -> ("BusNumberRef"=w301:refnum<vi>)
        n136 = call "RemoveBus.vi"("BusArray"=w303, "BusNumberRef"=w301, "BusNumber"=w297) -> ("BusArray"=w302:refnum<class "Bus.lvclass">[], "BusIndex"=w299:i32)  [unwired: 6 in]
        n137 = local read "QueName"() -> (w296:string)
        n138 = call "Enqueue.vi"("QueName"=w296, "Data"=w299, "Message"="RemoveBus") -> ("Error"=w300:errorcluster[])  [unwired: 8 in]
      }
      event User Event {
        # "Enabled?"
        n139 = event-data() -> ("ModuleID"=w309:i32, "Data"=w308:variant)  [unwired: 1 in]
        n140 = case shown="True" TRUE {
          tunnel: w310 -> [w311 w313]
          tunnel: w309 -> [_ w322]
          tunnel: w308 -> [_ w320]
          tunnel: [_ w317] -> w307
          tunnel: [w311 w313] -> w305
          frame False {
          }
          frame True {
            # "Find Bus Index"
            n141 = for {
              tunnel: w313 -> [w327] mode=indexing
              tunnel: w322 -> [w325]
              tunnel: [w323] -> w321
              i -> [w323]
              stop <- w324 stop-if-true
              n142 = property class="Bus.lvclass"(reference=w327) -> ("Accessors:EventModuleID"=w326:i32)  [unwired: 1 in, 2 out]
              n143 = Equal?(x=w326, y=w325) -> (x = y?=w324:bool)
            }
            n144 = Variant To Data(type=T3 [] ("clEvtReportArray"), Variant=w320) -> (data=w318:T3)  [unwired: 1 in, 1 out]
            n145 = Bundle By Name(cluster=T17 {"BusIndex"=0, "clImpairReportArray"=[]} ("clEvtReportArray"), "BusIndex"=w321, "clImpairReportArray"=w318) -> (w316:T17)
            n146 = local read "QueName"() -> (w312:string)
            n147 = call "Enqueue.vi"("QueName"=w312, "Data"=w316, "Message"="EventReport") -> ("Error"=w317:errorcluster[])  [unwired: 8 in]
          }
        }
      }
      event User Event {
        # "Enabled?"
        n148 = event-data() -> ("ModuleID"=w332:i32, "Data"=w331:variant)  [unwired: 1 in]
        n149 = case shown="True" TRUE {
          tunnel: w333 -> [w334 w336]
          tunnel: w332 -> [_ w345]
          tunnel: w331 -> [_ w343]
          tunnel: [_ w340] -> w330
          tunnel: [w334 w336] -> w328
          frame False {
          }
          frame True {
            # "Find Bus Index"
            n150 = for {
              tunnel: w336 -> [w350] mode=indexing
              tunnel: w345 -> [w348]
              tunnel: [w346] -> w344
              i -> [w346]
              stop <- w347 stop-if-true
              n151 = property class="Bus.lvclass"(reference=w350) -> ("Accessors:EventModuleID"=w349:i32)  [unwired: 1 in, 2 out]
              n152 = Equal?(x=w349, y=w348) -> (x = y?=w347:bool)
            }
            n153 = Variant To Data(type=T5 [] ("dblEventSignalArray"), Variant=w343) -> (data=w341:T5)  [unwired: 1 in, 1 out]
            n154 = Bundle By Name(cluster=T22 {"BusIndex"=0, "dblEventSignalArray"=[]} ("clEvtReportArray"), "BusIndex"=w344, "dblEventSignalArray"=w341) -> (w339:T22)
            n155 = local read "QueName"() -> (w335:string)
            n156 = call "Enqueue.vi"("QueName"=w335, "Data"=w339, "Message"="EventSignal") -> ("Error"=w340:errorcluster[])  [unwired: 8 in]
          }
        }
      }
      event User Event {
        # "Enabled?"
        n157 = event-data() -> ("ModuleID"=w356:i32, "Data"=w355:variant)  [unwired: 1 in]
        n158 = case shown="True" TRUE {
          tunnel: w357 -> [w358 w362]
          tunnel: w356 -> [_ w369]
          tunnel: w355 -> [_ w368]
          tunnel: [_ w360] -> w354
          tunnel: [w358 w362] -> w352
          tunnel: w351 -> [_ _]
          frame False {
          }
          frame True {
            # "Find Bus Index"
            n159 = for {
              tunnel: w362 -> [w374] mode=indexing
              tunnel: w369 -> [w372]
              tunnel: [w370] -> w361
              i -> [w370]
              stop <- w371 stop-if-true
              n160 = property class="Bus.lvclass"(reference=w374) -> ("Accessors:EventModuleID"=w373:i32)  [unwired: 1 in, 2 out]
              n161 = Equal?(x=w373, y=w372) -> (x = y?=w371:bool)
            }
            n162 = Variant To Data(type=T3 [] ("clEvtReportArray"), Variant=w368) -> (data=w366:T3)  [unwired: 1 in, 1 out]
            n163 = Bundle By Name(cluster=T18 {"BusIndex"=0, "clImpairReportArray"=[]} ("clEvtReportArray"), "BusIndex"=w361, "clImpairReportArray"=w366) -> (w365:T18)
            n164 = local read "QueName"() -> (w359:string)
            n165 = call "Enqueue.vi"("QueName"=w359, "Data"=w365, "Message"="PmuImpairRpt") -> ("Error"=w360:errorcluster[])  [unwired: 8 in]
          }
        }
      }
      event User Event {
        # "Enabled?"
        n166 = event-data() -> ("ModuleID"=w379:i32, "Data"=w378:variant)  [unwired: 1 in]
        n167 = case shown="True" FALSE {
          tunnel: w380 -> [w381 w383]
          tunnel: w379 -> [_ w392]
          tunnel: w378 -> [_ w390]
          tunnel: [_ w387] -> w377
          tunnel: [w381 w383] -> w375
          frame False {
          }
          frame True {
            # "Find Bus Index"
            n168 = for {
              tunnel: w383 -> [w397] mode=indexing
              tunnel: w392 -> [w395]
              tunnel: [w393] -> w391
              i -> [w393]
              stop <- w394 stop-if-true
              n169 = property class="Bus.lvclass"(reference=w397) -> ("Accessors:EventModuleID"=w396:i32)  [unwired: 1 in, 2 out]
              n170 = Equal?(x=w396, y=w395) -> (x = y?=w394:bool)
            }
            n171 = Variant To Data(type=T6 [] ("dblNetworkTime"), Variant=w390) -> (data=w388:T6)  [unwired: 1 in, 1 out]
            n172 = Bundle By Name(cluster=T19 {"BusIndex"=0, "clNetImpairTimeArray"=[]} ("clEvtReportArray"), "BusIndex"=w391, "clNetImpairTimeArray"=w388) -> (w386:T19)
            n173 = local read "QueName"() -> (w382:string)
            n174 = call "Enqueue.vi"("QueName"=w382, "Data"=w386, "Message"="NetImpairTime") -> ("Error"=w387:errorcluster[])  [unwired: 8 in]
          }
        }
      }
      event User Event {
        # "Enabled?"
        n175 = event-data() -> ("ModuleID"=w402:i32, "Data"=w401:variant)  [unwired: 1 in]
        n176 = case shown="True" FALSE {
          tunnel: w403 -> [w404 w406]
          tunnel: w402 -> [_ w415]
          tunnel: w401 -> [_ w413]
          tunnel: [_ w410] -> w400
          tunnel: [w404 w406] -> w398
          frame False {
          }
          frame True {
            # "Find Bus Index"
            n177 = for {
              tunnel: w406 -> [w420] mode=indexing
              tunnel: w415 -> [w418]
              tunnel: [w416] -> w414
              i -> [w416]
              stop <- w417 stop-if-true
              n178 = property class="Bus.lvclass"(reference=w420) -> ("Accessors:EventModuleID"=w419:i32)  [unwired: 1 in, 2 out]
              n179 = Equal?(x=w419, y=w418) -> (x = y?=w417:bool)
            }
            n180 = Variant To Data(type=T7 [] ("dblPktLoss"), Variant=w413) -> (data=w411:T7)  [unwired: 1 in, 1 out]
            n181 = Bundle By Name(cluster=T20 {"BusIndex"=0, "clNetPktLoss"=[]} ("clEvtReportArray"), "BusIndex"=w414, "clNetPktLoss"=w411) -> (w409:T20)
            n182 = local read "QueName"() -> (w405:string)
            n183 = call "Enqueue.vi"("QueName"=w405, "Data"=w409, "Message"="NetPktLoss") -> ("Error"=w410:errorcluster[])  [unwired: 8 in]
          }
        }
      }
      event User Event {
        # "Enabled?"
        n184 = event-data() -> ("ModuleID"=w425:i32, "Data"=w424:variant)  [unwired: 1 in]
        n185 = case shown="True" FALSE {
          tunnel: w426 -> [w427 w429]
          tunnel: w425 -> [_ w438]
          tunnel: w424 -> [_ w436]
          tunnel: [_ w433] -> w423
          tunnel: [w427 w429] -> w421
          frame False {
          }
          frame True {
            # "Find Bus Index"
            n186 = for {
              tunnel: w429 -> [w443] mode=indexing
              tunnel: w438 -> [w441]
              tunnel: [w439] -> w437
              i -> [w439]
              stop <- w440 stop-if-true
              n187 = property class="Bus.lvclass"(reference=w443) -> ("Accessors:EventModuleID"=w442:i32)  [unwired: 1 in, 2 out]
              n188 = Equal?(x=w442, y=w441) -> (x = y?=w440:bool)
            }
            n189 = Variant To Data(type=T8 [] ("ui32FlagImpairmentArray"), Variant=w436) -> (data=w434:T8)  [unwired: 1 in, 1 out]
            n190 = Bundle By Name(cluster=T21 {"BusIndex"=0, "FlagImpairArray"=[]} ("clEvtReportArray"), "BusIndex"=w437, "FlagImpairArray"=w434) -> (w432:T21)
            n191 = local read "QueName"() -> (w428:string)
            n192 = call "Enqueue.vi"("QueName"=w428, "Data"=w432, "Message"="FlagImpair") -> ("Error"=w433:errorcluster[])  [unwired: 8 in]
          }
        }
      }
      event User Event {
        n193 = event-data() -> ()  [unwired: 1 in, 1 out]
        n194 = local read "QueName"() -> (w444:string)
        n195 = call "Enqueue.vi"("QueName"=w444, "Priority? (F)"=TRUE, "Message"="Stop") -> ("Error"=w448:errorcluster[])  [unwired: 8 in]
      }
      event "btnStop": Value Change {
        n196 = event-data() -> ()  [unwired: 1 in, 1 out]
        n197 = call "ObtainRequestEvents.vi"() -> ("Error"=w460:errorcluster[], "clRequestEvents"=w457:T9)  [unwired: 10 in]
        n198 = Unbundle By Name(w457) -> ("StopRequest"=w458:refnum<user-event>)
        n199 = Generate User Event(priority (normal)=usereventprio."high priority", user event=w458, event data cluster=T23 {"BusIndex"=0, "Data"=variant} ("event data")) -> (error out=w459:errorcluster)  [unwired: 1 in, 1 out]
        n200 = call <userlib>:"AddError.vi"("Severity"="Fatal" ("String"), "Priority"=u8 0, "ErrorArray"=w460, "error in (no error)"=w459) -> ("ErrorArray"=w456:errorcluster[], "error out"=w453:errorcluster)  [unwired: 6 in]
        n201 = call <vilib>:"Clear Errors.vi"("error in (no error)"=w453) -> ()  [unwired: 5 in, 2 out]
      }
    }
    n202 = local read "QueName"() -> (w257:string)
    n203 = call "EnqueError.vi"("QueName"=w257, "Error"=w262) -> ("Error"=w261:errorcluster[])  [unwired: 9 in]
  }
  n204 = Build Array (concatenate)(w30, w31) -> (w1:errorcluster[])
  "ErrorArray" <- w1
  n205 = Empty Array?(array=w1) -> (empty?=w2:bool)
  n206 = case shown="True" w2 {
    frame False {
    }
    frame True {
      n207 = Current VI's Path() -> (path=w463:path)
      n208 = Build Path(base path=w463, name or relative path=path "../VisualizePMU.vi") -> (appended path=w461:path)
      n209 = Open VI Reference(vi path=w461) -> (vi reference=w464:refnum<vi>)  [unwired: 5 in, 1 out]
      n210 = invoke class="VI" method="FP.Close"(reference=w464) -> ()  [unwired: 2 in, 3 out]
    }
  }
